vi "5-1-1 delay imposto.vi"(1 "error in":bool, 2 "delay":u32=500) -> (0 "error out":bool)   [LabVIEW 2012]
doc: "© Copyright M. Ferrari 2000\n Delay function"
panel:
  # "[ms]"
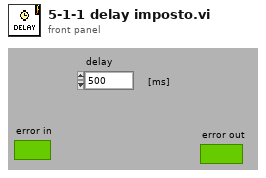
[diagram p1: front panel]
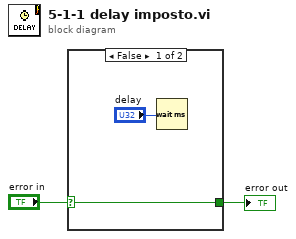
[diagram p0: block diagram]
diagram:
  n1 = case shown="False" "error in" {
    selector: "error in" -> [w4 w5]
    tunnel: [w4 w5] -> w1
    frame False {
      n2 = Wait (ms)(milliseconds to wait="delay") -> ()  [unwired: 1 out]
    }
    frame True {
    }
  }
  "error out" <- w1
